vi "Configure Ramp Symmetry.vi"(8 "error in (no error)":errorcluster, 10 "Ramp Symmetry (50%)":dbl=50.0 min=0.0 max=100.0 step=1.0 format="%.2f", 11 "VISA resource name":refnum<visa-resource-name>) -> (0 "error out":errorcluster, 3 "VISA resource name out":refnum<visa-resource-name>)   [LabVIEW 2017, in "Agilent 33XXX Series.lvlib"]
doc: "Configures the ramp symmetry for Ramp waveforms.\n\nNote:\n(1) This VI is only used with Agilent 33210A, 33220A and 33250A."
uses:
  Agilent 33XXX Series.lvlib
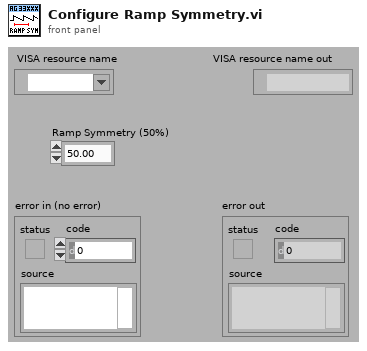
[diagram p1: front panel]
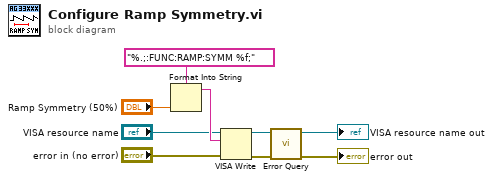
[diagram p0: block diagram]
diagram:
  n1 = Format Into String(format string="%.;:FUNC:RAMP:SYMM %f;", "Ramp Symmetry (50%)") -> (resulting string=w7:string)  [unwired: 2 in, 1 out]
  n2 = VISA Write(VISA resource name="VISA resource name", write buffer=w7, error in (no error)="error in (no error)") -> (VISA resource name out=w6:refnum<visa-resource-name>, error out=w5:errorcluster)  [unwired: 1 out]
  n3 = call "Error Query.vi"("error in (no error)"=w5, "VISA resource name"=w6) -> ("error out"=→"error out":errorcluster, "VISA resource name out"=→"VISA resource name out":refnum<visa-resource-name>)  [unwired: 6 in, 2 out]
